vi "To48BitSetting.vi"(10 "48 bit value":fxp<+,48,48>, 11 "FPGA Setting":T1=enum."Cavity C3") -> (3 "value":u64)   [LabVIEW 2018]
uses:
  FPGA/fpga_settings.ctl
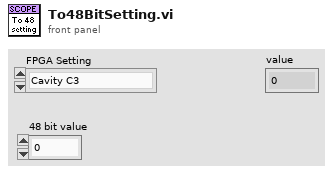
[diagram p1: front panel]
types:
  T1 = typedef "fpga_settings.ctl" = enum16{"Feedback Enable", "New FIR coeffs", "FIR shift", "Enable filter", "Set Downsample", "Downsample", "CIC Gain", "Record length", "Trigger samples", "Quiet time", "a_am", "b_am", "Use fixed delay", "fixed sin_fi", "fixed cos_fi", "Ki*Tau", "Kp", "Kd_Tau", "Fi_start", "Fi_delta", "DC_offs 0", "DC_offs 1", "DC_offs 2", "DC_offs 3", "Ki*Tau am", "Kp am", "Kd_Tau am", "Feedback AM", "Trigger delay", "Feedback delay", "Setpoint enable", "Beam enable", "Samples to acquire", "Cavity Enable", "Cavity C1", "Cavity C2", "Cavity C3", "Cavity C4", "Cavity C5", "Input delay", "Ki*Tau Q", "Kp Q", "Kd_Tau Q", "Adaptive FF enable", "Feedforward a0", "Feedforward b0", "FF src adress", "FF dest adress", "Output scale", "Input scale", "Host scale", "FF_IIR b0", "FF_IIR b1", "FF_IIR b2", "FF_IIR-a1", "FF_IIR-a2", "Enable HW trigger", "Virtual cavity", "Samples to skip", "Samples to skip 2", "Samples to skip 3"}
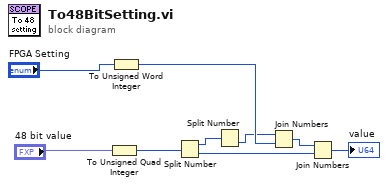
[diagram p0: block diagram]
diagram:
  n1 = To Unsigned Quad Integer(1:"48 bit value") -> (0:w8:u64)
  n2 = To Unsigned Word Integer(number="FPGA Setting") -> (unsigned 16bit integer=w6:u16)
  n3 = Split Number(x=w8) -> (hi(x)=w7:u32, lo(x)=w3:u32)
  n4 = Split Number(x=w7) -> (lo(x)=w5:u16)  [unwired: 1 out]
  n5 = Join Numbers(hi=w5, lo=w6) -> ((hi.lo)=w4:u32)
  n6 = Join Numbers(hi=w4, lo=w3) -> ((hi.lo)=→"value":u64)
